vi "I2CLCD1602.vi"() -> ()   [LabVIEW 2024]
uses:
  Driver/Public/I2C Options.ctl
  b9c42029-5a29-40f5-8131-c7213e8fe911.vi
  Driver/CTIPicoVISA.lvlib
panel:
  in  "Grove Connector":enum16{"I2C0", "I2C1"}(ring)
  in  "String 2":string="hello"
  out "Identity":T1
  in  "String":string="hello"
  out "error out":errorcluster={"status"=TRUE, "code"=15, "source"="CTI.lvlib:Session.lvclass:Check I2C Pins.vi:4130001<ERR>\nInvalid pin selection for I2C:\nGPIO 5 is invalid for I2C 1 SCL, valid options: 3, 7, 11, 15, 19, 27\r\nGPIO 4 is invalid for I2C 1 SDA, valid options: 2, 6, 10, 14, 18, 26\n\n\n<b>Complete call chain:</b>\r\n     CTI.lvlib:Session.lvclass:Check I2C Pins.vi:4130001\r\n     CTI.lvlib:Session.lvclass:Reserve I2C.vi\r\n     CTI.lvlib:Session.lvclass:Configure I2C.vi:7080001\r\n     I2CLCD1602.vi"}
  in  "Port":refnum<visa-resource-name>="COM7"
  # "https://www.seeedstudio.com/Grove-LCD-RGB-Backlight.html"
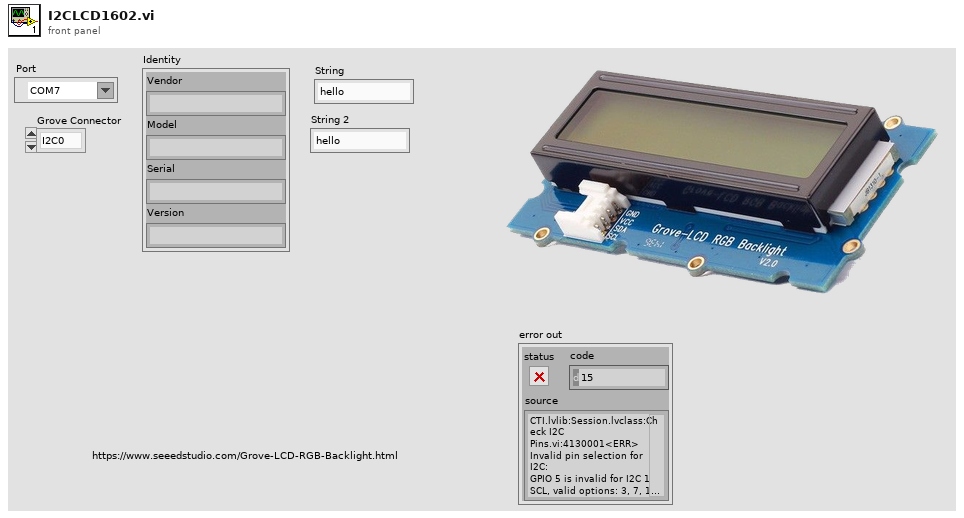
[diagram p1: front panel]
types:
  T1 = cluster{"Vendor":string, "Model":string, "Serial":string, "Version":string}
  T2 = typedef "CTIPicoVISA.lvlib/I2C Options.ctl" = cluster{"Baud":u32, "SCL GPIO":i32, "SDA GPIO":i32}
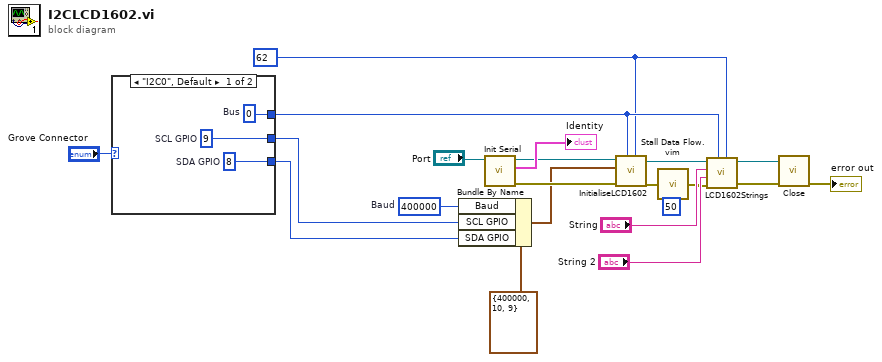
[diagram p0: block diagram]
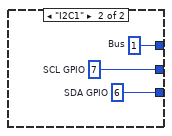
[diagram p2: hidden frame]
diagram:
  w3 = u8 62 ("Address")
  w9 = u32 400000  # Baud
  n1 = case shown="\"I2C0\", Default" "Grove Connector" {
    tunnel: [w24 w27] -> w8
    tunnel: [w23 w26] -> w7
    tunnel: [w22 w25] -> w4
    frame "I2C0", Default {
      w22 = u8 0  # Bus
      w23 = 8  # SDA GPIO
      w24 = 9  # SCL GPIO
    }
    frame "I2C1" {
      w25 = u8 1  # Bus
      w26 = 6  # SDA GPIO
      w27 = 7  # SCL GPIO
    }
  }
  n2 = Bundle By Name(cluster=T2 {"Baud"=400000, "SCL GPIO"=10, "SDA GPIO"=9} ("I2C Options"), "Baud"=w9, "SCL GPIO"=w8, "SDA GPIO"=w7) -> (w5:T2)
  n3 = call "Init Serial.vi"("VISA resource name in"="Port") -> ("error out"=w18:errorcluster, "Identity"=→"Identity":T1, "VISA resource name Out"=w19:refnum<visa-resource-name>)  [unwired: 8 in]
  n4 = call "InitialiseLCD1602.vi"("Address"=w3, "Bus"=w4, "error in (no error)"=w18, "I2C Options"=w5, "Port"=w19) -> ("error out"=w16:errorcluster, "VISA resource name"=w17:refnum<visa-resource-name>)  [unwired: 5 in]
  n5 = call "Stall Data Flow.vim"("value in"=w16, "milliseconds to wait"=u32 50) -> ("value out"=w2:errorcluster)  [unwired: 1 out]
  n6 = call "LCD1602Strings.vi"("Address"=w3, "Bus"=w4, "error in (no error)"=w2, "String 2"="String 2", "String"="String", "Port"=w17) -> ("error out"=w14:errorcluster, "VISA resource name"=w15:refnum<visa-resource-name>)  [unwired: 4 in]
  n7 = call "Close.vi"("error in (no error)"=w14, "VISA resource name in"=w15) -> ("error out"=→"error out":errorcluster)  [unwired: 9 in]
